vi "testStreamWriter.vi"(8 "error in (no error)":errorcluster, 11 "TestCase in":refnum<class "TestdotNetStreams.lvclass">) -> (0 "error out":errorcluster, 3 "TestCase out":refnum<class "TestdotNetStreams.lvclass">)   [LabVIEW 2021, in "TestdotNetStreams.lvclass"]
uses:
  TestdotNetStreams.lvclass
  <vilib>/addons/_JKI Toolkits/VI Tester/TestCase.llb/TestCase.lvclass
  C:/Program Files (x86)/National Instruments/LabVIEW 2021/vi.lib/addons/_JKI Toolkits/VI Tester/TestCase.llb/TestCase.lvclass
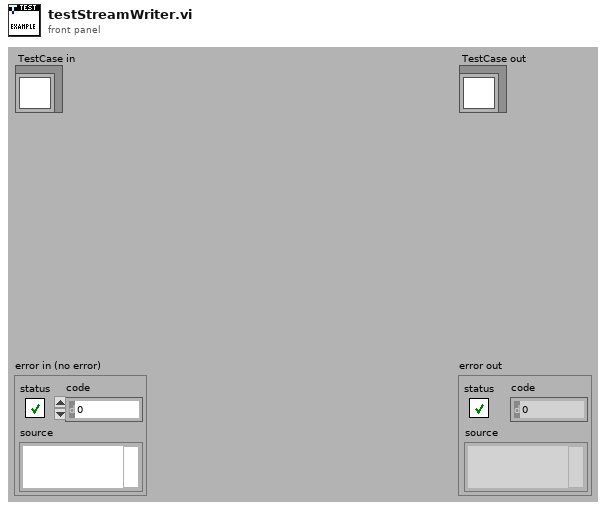
[diagram p1: front panel]
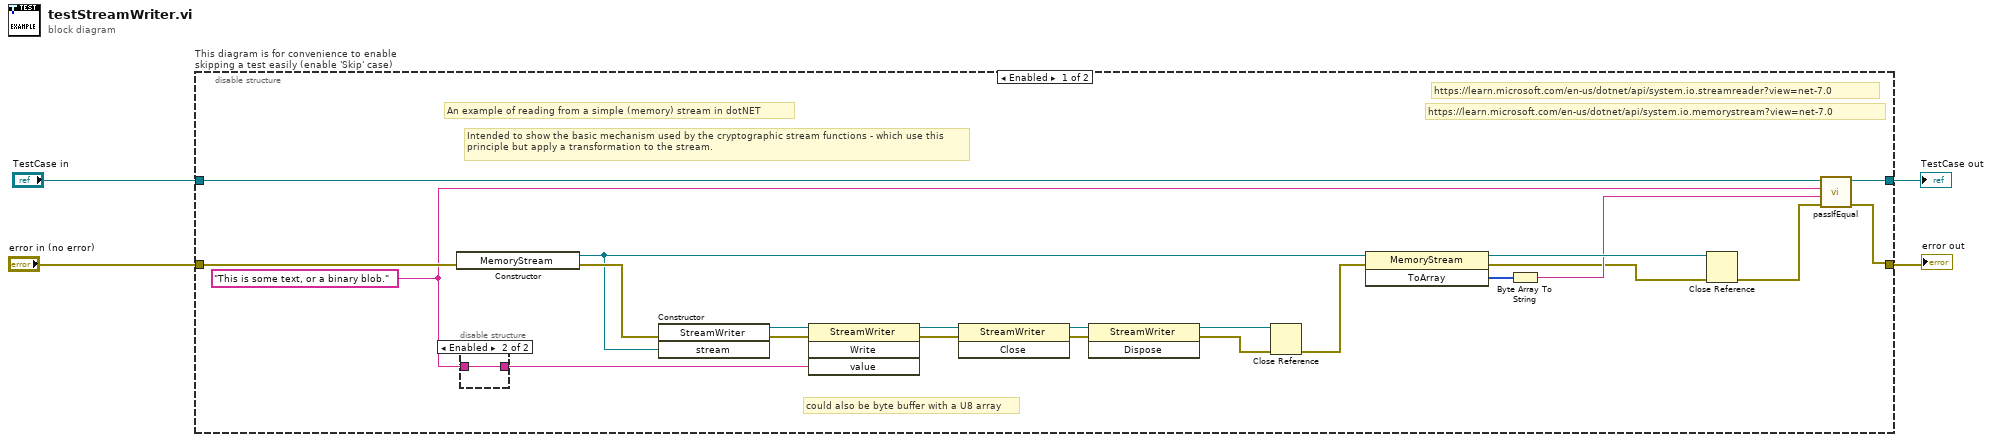
[diagram p0: block diagram]
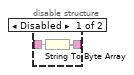
[diagram p2: hidden frame]
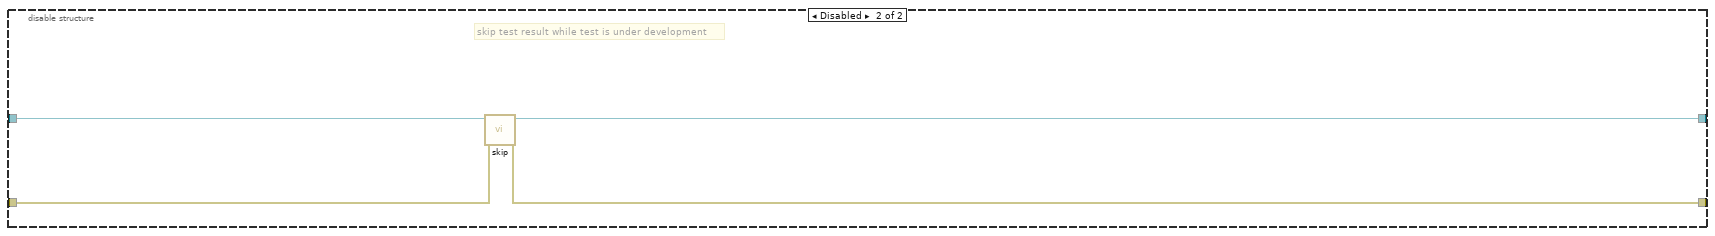
[diagram p3: hidden frame]
diagram:
  n1 = disable-structure "This diagram is for convenience to enable skipping a test easily (enable 'Skip' case)" shown="Enabled" {
    disable-tunnel: "TestCase in" -> [w26 w33]
    disable-tunnel: [w25 w31] -> w1
    disable-tunnel: [w24 w32] -> w3
    disable-tunnel: "error in (no error)" -> [w21 w30]
    frame Enabled {
      w16 = "This is some text, or a binary blob."
      # "could also be byte buffer with a U8 array"
      # "https://learn.microsoft.com/en-us/dotnet/api/system.io.memorystream?view=net-7.0"
      # "https://learn.microsoft.com/en-us/dotnet/api/system.io.streamreader?view=net-7.0"
      # "Intended to show the basic mechanism used by the cryptographic stream functions - which use this principle but apply a transformation to the stream."
      # "An example of reading from a simple (memory) stream in dotNET"
      n2 = constructor class="MemoryStream"(error in=w21) -> (reference out=w14:refnum<k24>, error out=w20:errorcluster)  [unwired: 2 in, 1 out]
      n3 = disable-structure shown="Enabled" {
        disable-tunnel: w16 -> [w28 w29]
        disable-tunnel: [w27 w29] -> w15
        frame Disabled {
          n4 = String To Byte Array(string=w28) -> (unsigned byte array=w27:u8[])
        }
        frame Enabled {
        }
      }
      n5 = constructor class="StreamWriter"(error in=w20, "stream"=w14) -> (reference out=w23:refnum<k24>, error out=w22:errorcluster)  [unwired: 2 in, 2 out]
      n6 = invoke class="StreamWriter" method="Write"(reference=w23, error in=w22, "value"=w15) -> (reference out=w10:refnum<k24>, error out=w9:errorcluster)  [unwired: 1 in, 2 out]
      n7 = invoke class="StreamWriter" method="Close"(reference=w10, error in=w9) -> (reference out=w7:refnum<k24>, error out=w8:errorcluster)  [unwired: 1 in, 1 out]
      n8 = invoke class="StreamWriter" method="Dispose"(reference=w7, error in=w8) -> (reference out=w17:refnum<k24>, error out=w18:errorcluster)  [unwired: 1 in, 1 out]
      n9 = Close Reference(reference=w17, error in (no error)=w18) -> (error out=w6:errorcluster)
      n10 = invoke class="MemoryStream" method="ToArray"(reference=w14, error in=w6) -> (reference out=w13:refnum<k24>, error out=w5:errorcluster, "ToArray"=w12:u8[])  [unwired: 1 in]
      n11 = Byte Array To String(unsigned byte array=w12) -> (string=w11:string)
      n12 = Close Reference(reference=w13, error in (no error)=w5) -> (error out=w19:errorcluster)
      n13 = call-dynamic "passIfEqual.vi"("error in (no error)"=w19, "y"=w11, "x"=w16, "TestCase in"=w26) -> ("error out"=w24:errorcluster, "TestCase out"=w25:refnum<class "TestdotNetStreams.lvclass">)  [unwired: 6 in]
    }
    frame Disabled {
      # "skip test result while test is under development"
      n14 = call <vilib>:"skip.vi"("error in (no error)"=w30, "TestCase in"=w33) -> ("error out"=w32:errorcluster, "TestCase out"=w31:refnum<class "TestdotNetStreams.lvclass">)  [unwired: 8 in]
    }
  }
  "error out" <- w3
  "TestCase out" <- w1
